vi "LDA_BSA_Comms_F60.vi"(2 "LDA Channels":T1[](array[typedef]) {"Sync Delay (s)" format="%.2g"; "Req Sampling Rate Hz" min=1.0; "Shifted mW" format="%.1g"; "Unshifted mW" format="%.1g"; "Centre Velocity (m/s)" format="%.2g"; "Velocity Range (m/s)" format="%.2g"; "Focal Length (mm)" format="%.1f"; "Beam Separation (mm)" format="%.1f"; "Optics Conversion Factor" format="%.3g"; "High voltage" min=0 max=2040 step=8; "Signal gain (dB)" min=0 max=30 step=1; "Min Velocity" format="%.2g"; "Max Velocity" format="%.2g"; "Wavelength (nm)" format="%.1f"}, 3 "BSA":refnum<k7>) -> (0 "error out":errorcluster, 1 "LDA Raw Data":cluster{dbl[][]}[](array[cluster]))   [LabVIEW 2021]
uses:
  LDA_Channel.ctl
  Globals/Meas_global.vi
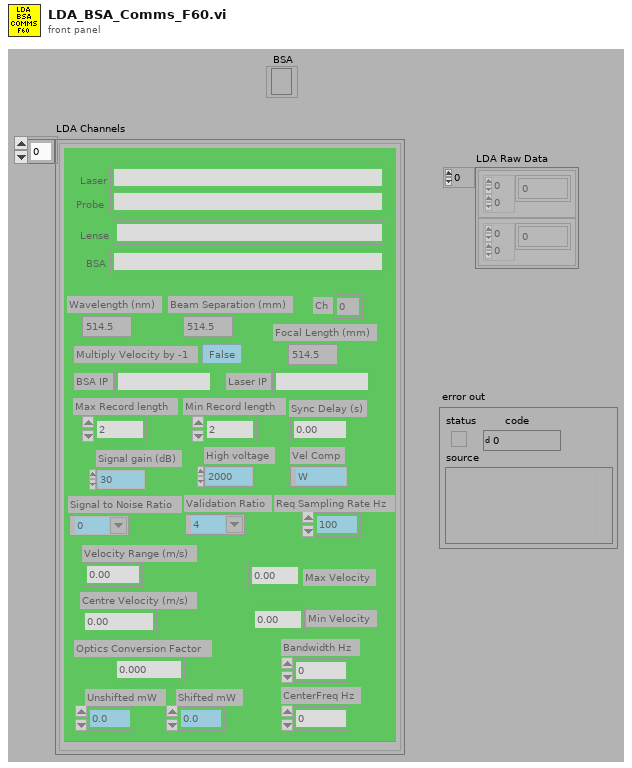
[diagram p1: front panel]
types:
  T1 = typedef "LDA_Channel.ctl" = cluster{"Wavelength (nm)":dbl, "Vel Comp":string, "Max Velocity":dbl, "Min Velocity":dbl, "Max Record length":u16, "Signal gain (dB)":i16, "High voltage":i16, "Optics Conversion Factor":dbl, "Min Record length":u16, "Multiply Velocity by -1":bool, "Signal to Noise Ratio":string, "Validation Ratio":string, "Probe":string, "Laser":string, "BSA":string, "Lense":string, "Beam Separation (mm)":dbl, "Focal Length (mm)":dbl, "COLOUR":u32, "BSA IP":string, "Velocity Range (m/s)":dbl, "Centre Velocity (m/s)":dbl, "Unshifted mW":dbl, "Shifted mW":dbl, "Bandwidth Hz":dbl, "Req Sampling Rate Hz":dbl, "Ch":i32, "CenterFreq Hz":dbl, "Laser IP":string, "Sync Delay (s)":dbl}
  T2 = typedef "Analysis_info_cluster.ctl" = cluster{"Colour":u32, "Inst type":T3, "Inst name":string, "Symbol":string, "Code name":string, "Extra Info":string, "Inst Array":T4, "Extra Titles":string[], "Extra Values":string[], "U":dbl, "u^2":dbl, "u^3":dbl, "u^4":dbl, "Skew_u":dbl, "Kurt_u":dbl, "Sd Error in Mean":dbl, "% u'/U":dbl, "X":dbl, "Y":dbl, "Z":dbl, "Timescale integral Estimate":dbl, "Sd Error in Variance":dbl, "Calib File":path, "Calib Constants":dbl[], "Output Position":bool, "Stats":enum16{"None", "Basic", "Full"}, "Av Sampling Rate":dbl, "Av No of Samples":dbl, "Total Meas Time (s)":dbl, "ADAM Ch Name":string, "Max value":dbl, "Min value":dbl, "Req Sample Rate Hz":dbl, "Sync Delay Time (s)":dbl, "Ch No":i16, "Device":string, "Use Latest Calib":bool, "Port":string, "Metadata Ch Names":string[], "Metadata Ch Values":string[], "Label":string}
  T3 = typedef "Inst_type.ctl" = enum16{"Raw voltage", "Raw with zero offsetting", "Propeller anemometer", "Pressure Transducer", "Pitot-static tube", "Hot wire", "Cross wire 1", "Cross wire 2", "Generic Linear", "Generic Polynomial", "Generic BackPoly", "Fast FID", "Thermocouple", "Cold wire", "Pulsed Wire", "LDA Vel", "LDA Tran time", "LDA Arr time", "Microphone"}
  T4 = typedef "Instrument_Array.ctl" = enum16{"PWA", "LDA", "Analogue"}
  T5 = typedef "Trigger_Mode.ctl" = enum16{"Free Running", "Start on Trigger", "Trigger Every Block", "Trigger Every Sample"}
  T6 = typedef "Rendezvous RefNum" = refnum<k1>
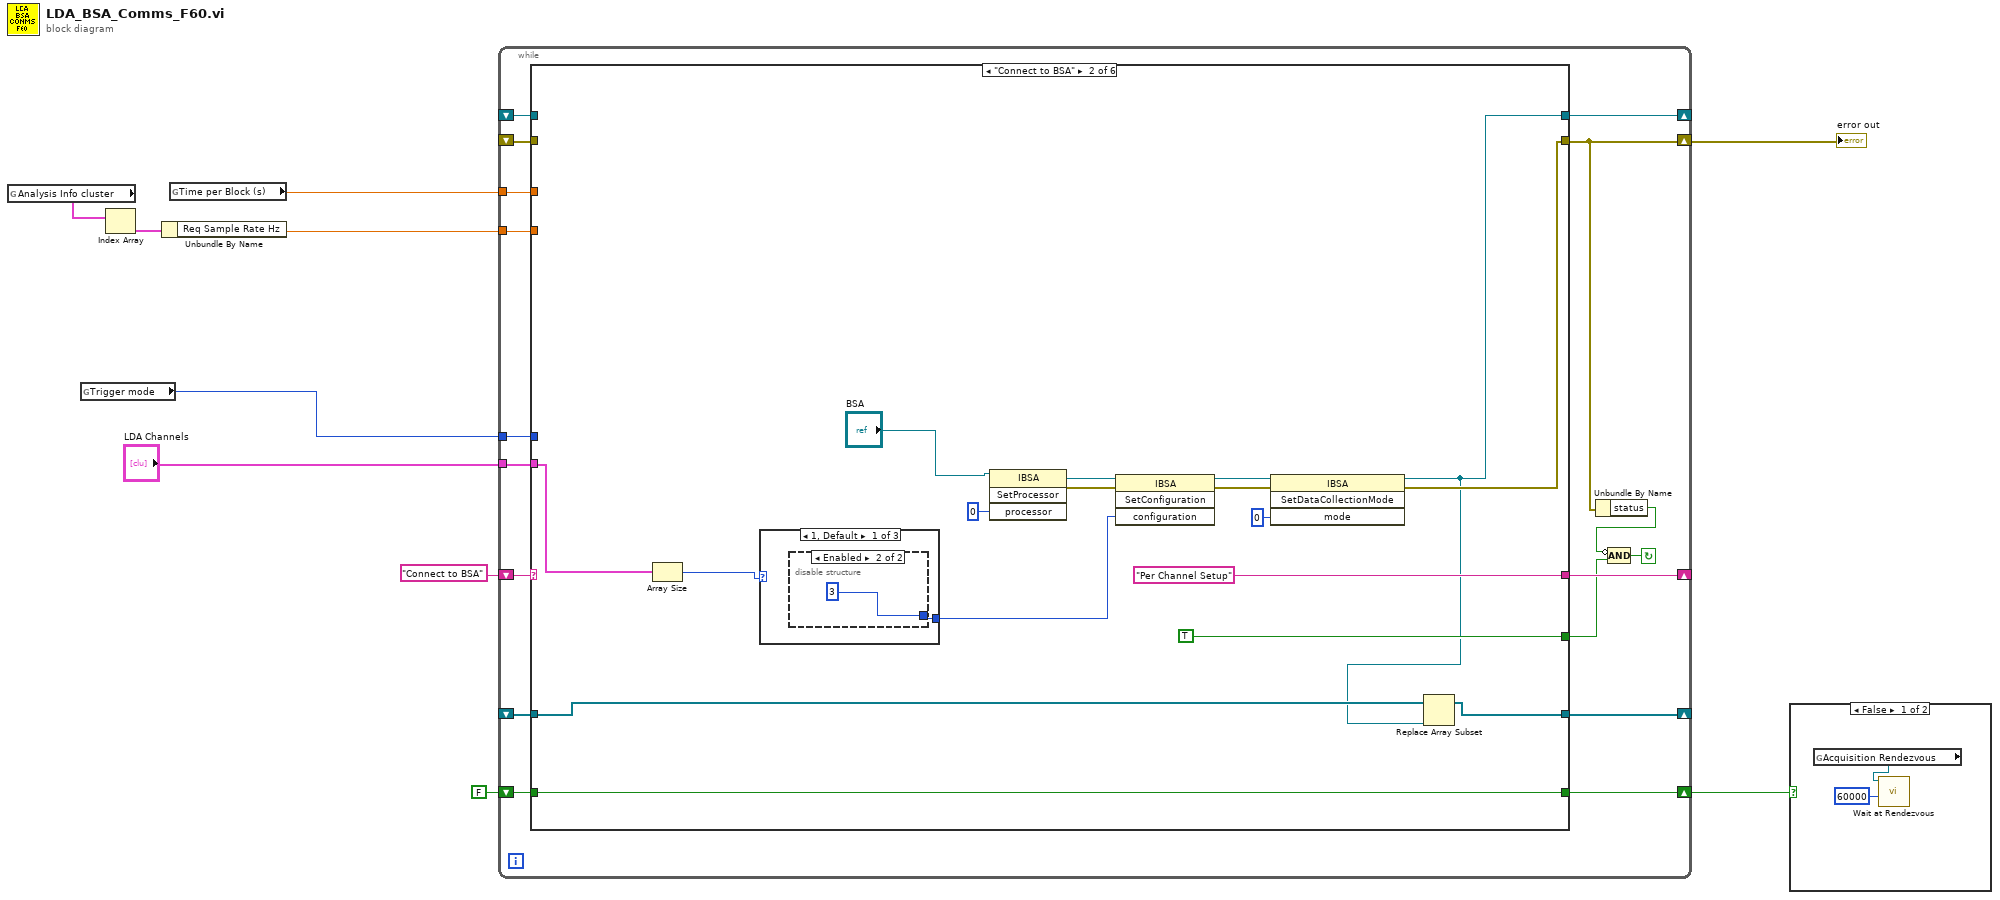
[diagram p0: block diagram]
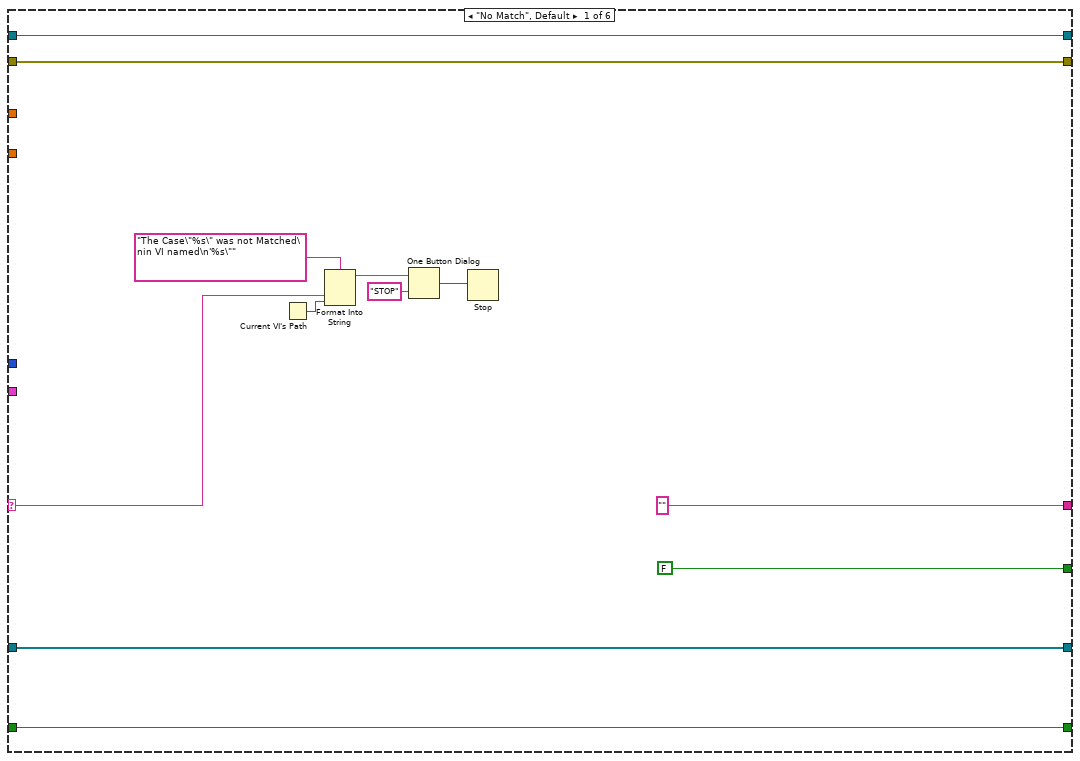
[diagram p2: hidden frame]
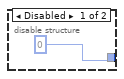
[diagram p3: hidden frame]
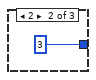
[diagram p4: hidden frame]
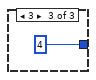
[diagram p5: hidden frame]
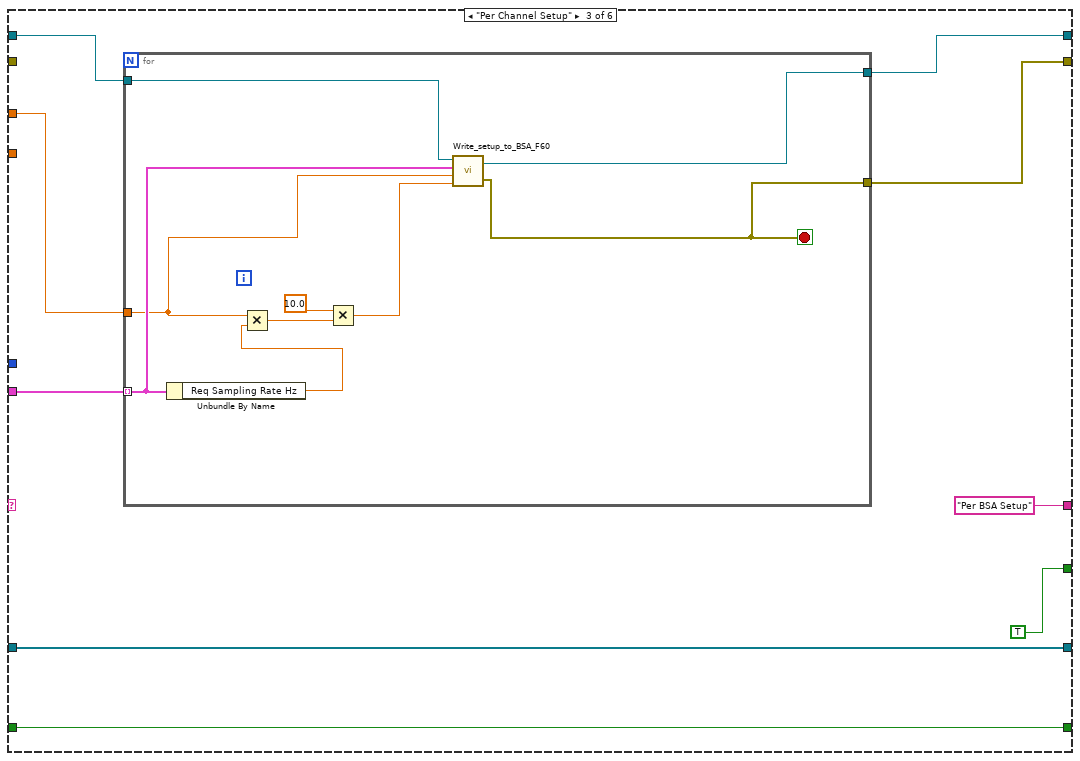
[diagram p6: hidden frame]
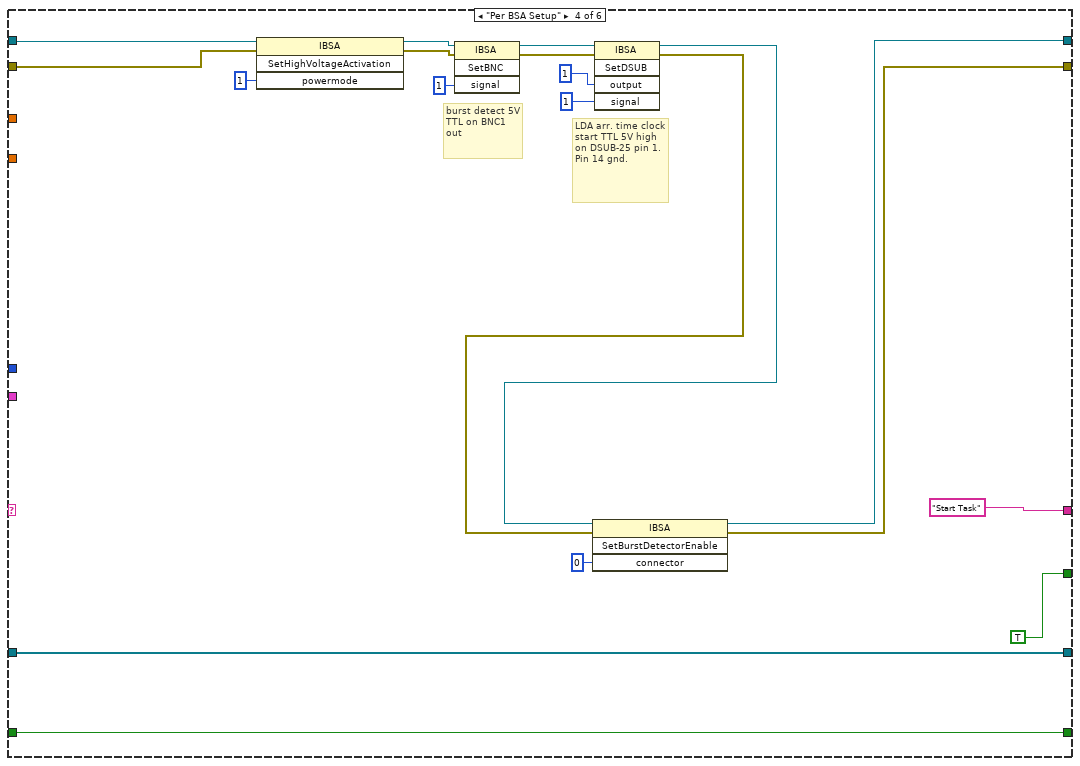
[diagram p7: hidden frame]
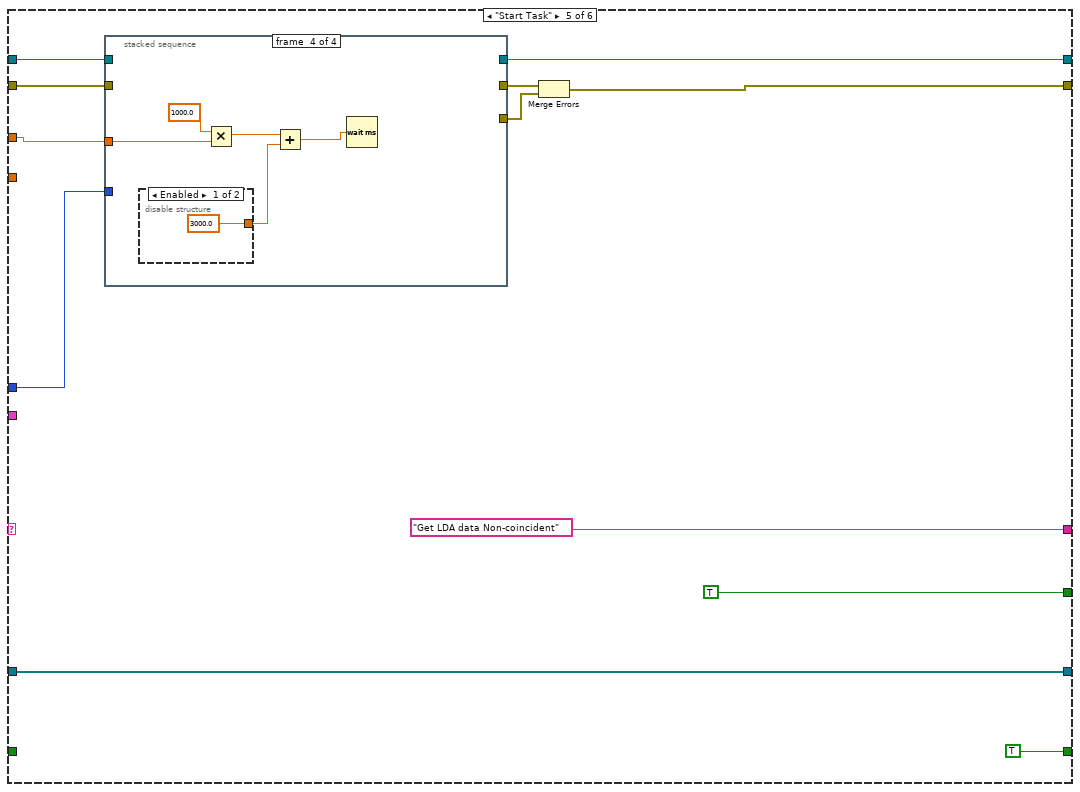
[diagram p8: hidden frame]
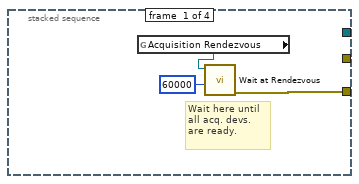
[diagram p9: hidden frame]
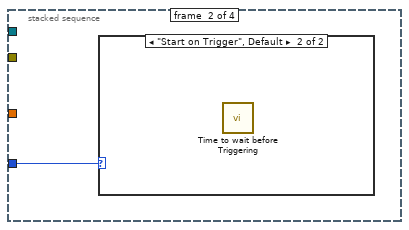
[diagram p10: hidden frame]
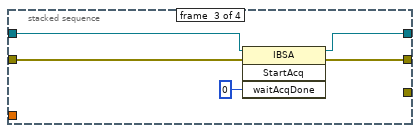
[diagram p12: hidden frame]
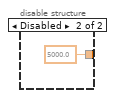
[diagram p13: hidden frame]
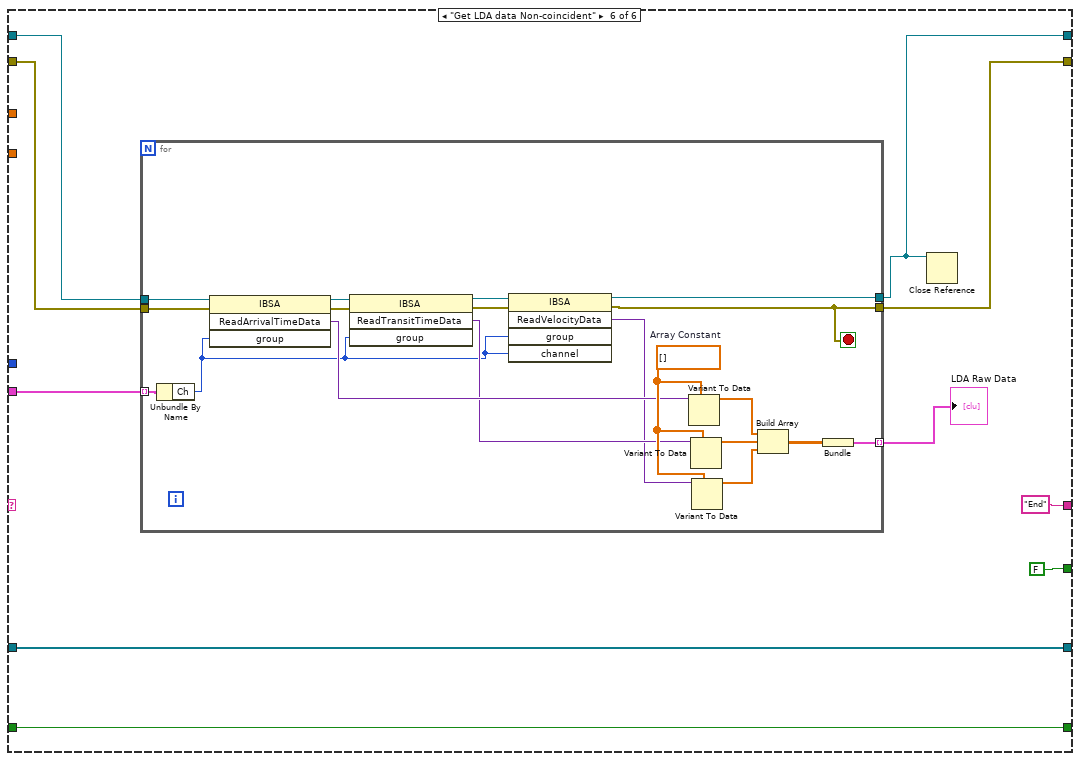
[diagram p14: hidden frame]
diagram:
  n1 = global read "Meas_global.vi" "Analysis Info cluster"() -> (w9:T2[])
  n2 = global read "Meas_global.vi" "Trigger mode"() -> (w5:T5)
  n3 = Index Array(array=w9) -> (element=w8:T2)  [unwired: 1 in]
  n4 = Unbundle By Name(w8) -> ("Req Sample Rate Hz"=w7:dbl)
  n5 = global read "Meas_global.vi" "Time per Block (s)"() -> (w6:dbl)
  n6 = while {
    shift-left: "Connect to BSA" -> [w26]
    shift-right: [w27] -> _
    shift-right: [w23] -> w10
    shift-left: _ -> [w16]
    tunnel: w7 -> [w25]
    shift-right: [w24] -> _
    shift-left: _ -> [w17]
    tunnel: w6 -> [w19]
    tunnel: w5 -> [w18]
    tunnel: "LDA Channels" -> [w15]
    shift-right: [w14] -> w4
    shift-left: FALSE -> [w13]
    shift-right: [w11] -> _
    shift-left: _ -> [w12]
    stop <- w21 continue-if-true
    n7 = case shown="\"Connect to BSA\"" w26 {
      selector: w26 -> [w30 _ _ _ _ _]
      tunnel: [FALSE TRUE TRUE TRUE TRUE FALSE] -> w20
      tunnel: ["" "Per Channel Setup" "Per BSA Setup" "Start Task" "Get LDA data Non-coincident" "End"] -> w27
      tunnel: [w32 w48 w64 w93 w105 w132] -> w23
      tunnel: w16 -> [w32 _ _ w96 w103 w135]
      tunnel: w25 -> [_ _ _ _ _ _]
      tunnel: w17 -> [w31 _ w66 w97 w104 w136]
      tunnel: [w31 w45 w65 w94 w109 w127] -> w24
      tunnel: w19 -> [_ _ w69 _ w99 _]
      tunnel: w18 -> [_ _ _ _ w102 _]
      tunnel: w15 -> [_ w42 w67 _ _ w131]
      tunnel: [w29 w47 w63 w81 TRUE w130] -> w14
      tunnel: w13 -> [w29 w47 w63 w81 _ w130]
      tunnel: w12 -> [w28 w46 w62 w80 w100 w129]
      tunnel: [w28 w44 w62 w80 w100 w129] -> w11
      frame "No Match", Default {
        n8 = Current VI's Path() -> (path=w34:path)
        n9 = Format Into String(format string="The Case\"%s\" was not Matched\nin VI named\n'%s\"" ("Format String"), w30, w34) -> (resulting string=w37:string)  [unwired: 2 in, 1 out]
        n10 = One Button Dialog(message=w37, button name ("OK")="STOP") -> (true=w35:bool)
        n11 = Stop(stop? (T)=w35) -> ()
      }
      frame "Connect to BSA" {
        n12 = Array Size(array=w42) -> (size(s)=w41:i32)
        n13 = case shown="1, Default" w41 {
          tunnel: [w57 3 ("configuration") 4 ("configuration")] -> w40
          frame 1, Default {
            n14 = disable-structure shown="Enabled" {
              disable-tunnel: [0 ("configuration") 3 ("configuration")] -> w57
              frame Disabled {
              }
              frame Enabled {
              }
            }
          }
          frame 2 {
          }
          frame 3 {
          }
        }
        n15 = invoke class="IBSA" method="SetProcessor"(reference="BSA", "processor"=0) -> (reference out=w53:refnum<k7>, error out=w52:errorcluster)  [unwired: 2 in, 2 out]
        n16 = invoke class="IBSA" method="SetConfiguration"(reference=w53, error in=w52, "configuration"=w40) -> (reference out=w51:refnum<k7>, error out=w50:errorcluster)  [unwired: 1 in, 2 out]
        n17 = invoke class="IBSA" method="SetDataCollectionMode"(reference=w51, error in=w50, "mode"=0) -> (reference out=w45:refnum<k7>, error out=w48:errorcluster)  [unwired: 1 in, 2 out]
        n18 = Replace Array Subset(array=w46, new element=w45) -> (w44:refnum<k7>[])  [unwired: 1 in]
      }
      frame "Per Channel Setup" {
        n19 = for {
          tunnel: w69 -> [w74]
          tunnel: w67 -> [w75] mode=indexing
          tunnel: w66 -> [w76]
          tunnel: [w72] -> w65
          tunnel: [w71] -> w64
          stop <- w71 stop-if-true
          n20 = Unbundle By Name(w75) -> ("Req Sampling Rate Hz"=w77:dbl)
          n21 = Multiply(x=w74, y=w77) -> (x*y=w78:dbl)
          n22 = Multiply(x=10.0 ("y"), y=w78) -> (x*y=w73:dbl)
          n23 = call "Write_setup_to_BSA_F60.vi"("No Of Samples"=w73, "Time (s)"=w74, "BSA Setup In"=w75, "BSA"=w76) -> ("error out"=w71:errorcluster, "reference out"=w72:refnum<k7>)
        }
      }
      frame "Per BSA Setup" {
        # "LDA arr. time clock start TTL 5V high on DSUB-25 pin 1. Pin 14 gnd."
        # "burst detect 5V TTL on BNC1 out"
        n24 = invoke class="IBSA" method="SetHighVoltageActivation"(reference=w97, error in=w96, "powermode"=1) -> (reference out=w85:refnum<k7>, error out=w84:errorcluster)  [unwired: 1 in, 2 out]
        n25 = invoke class="IBSA" method="SetBNC"(reference=w85, error in=w84, "signal"=1) -> (reference out=w92:refnum<k7>, error out=w91:errorcluster)  [unwired: 1 in, 2 out]
        n26 = invoke class="IBSA" method="SetDSUB"(reference=w92, error in=w91, "output"=1 ("signal"), "signal"=1) -> (reference out=w83:refnum<k7>, error out=w82:errorcluster)  [unwired: 1 in, 3 out]
        n27 = invoke class="IBSA" method="SetBurstDetectorEnable"(reference=w83, error in=w82, "connector"=0) -> (reference out=w94:refnum<k7>, error out=w93:errorcluster)  [unwired: 1 in, 2 out]
      }
      frame "Start Task" {
        n28 = stacked-sequence {
          tunnel: [_ _ w116 _] -> w107
          tunnel: w104 -> [_ _ w117 _]
          tunnel: [_ _ w115 _] -> w109
          tunnel: w103 -> [_ _ w118 _]
          tunnel: [w112 _ _ _] -> w106
          tunnel: w102 -> [_ w114 _ _]
          tunnel: w99 -> [_ _ _ w124]
          frame #0 {
            # "Wait here until all acq. devs. are ready."
            n29 = global read "Meas_global.vi" "Acquisition Rendezvous"() -> (w113:T6)
            n30 = call <vilib>:"Wait at Rendezvous.vi"("ms timeout (-1)"=60000, "rendezvous"=w113) -> ("error out"=w112:errorcluster)  [unwired: 3 in, 2 out]
          }
          frame #1 {
            n31 = case shown="\"Start on Trigger\", Default" w114 {
              frame "Free Running" {
              }
              frame "Start on Trigger", Default {
                n32 = call "Time to wait before Triggering.vi"() -> ()  [unwired: 12 in]
              }
            }
          }
          frame #2 {
            n33 = invoke class="IBSA" method="StartAcq"(reference=w117, error in=w118, "waitAcqDone"=0) -> (reference out=w115:refnum<k7>, error out=w116:errorcluster)  [unwired: 1 in, 2 out]
          }
          frame #3 {
            n34 = disable-structure shown="Enabled" {
              disable-tunnel: [3000.0 ("y") 5000.0 ("y")] -> w121
              frame Enabled {
              }
              frame Disabled {
              }
            }
            n35 = Multiply(x=1000.0, y=w124) -> (x*y=w122:dbl)
            n36 = Add(x=w122, y=w121) -> (x+y=w120:dbl)
            n37 = Wait (ms)(milliseconds to wait=w120) -> ()  [unwired: 1 out]
          }
        }
        n38 = Merge Errors(w107, w106) -> (w105:errorcluster)
      }
      frame "Get LDA data Non-coincident" {
        n39 = for {
          tunnel: w136 -> [w147]
          tunnel: w135 -> [w146]
          tunnel: [w141] -> w128 mode=indexing
          tunnel: [w140] -> w127
          tunnel: [w139] -> w132
          tunnel: w131 -> [w138] mode=indexing
          stop <- w139 stop-if-true
          w151 = dbl[] []  # Array Constant
          n40 = Unbundle By Name(w138) -> ("Ch"=w137:i32)
          n41 = invoke class="IBSA" method="ReadArrivalTimeData"(reference=w147, error in=w146, "group"=w137) -> (reference out=w155:refnum<k7>, error out=w154:errorcluster, "ReadArrivalTimeData"=w150:variant)  [unwired: 1 in, 1 out]
          n42 = invoke class="IBSA" method="ReadTransitTimeData"(reference=w155, error in=w154, "group"=w137) -> (reference out=w153:refnum<k7>, error out=w152:errorcluster, "ReadTransitTimeData"=w149:variant)  [unwired: 1 in, 1 out]
          n43 = invoke class="IBSA" method="ReadVelocityData"(reference=w153, error in=w152, "group"=w137, "channel"=w137) -> (reference out=w140:refnum<k7>, error out=w139:errorcluster, "ReadVelocityData"=w148:variant)  [unwired: 1 in, 2 out]
          n44 = Variant To Data(type=w151, Variant=w150) -> (data=w145:dbl[])  [unwired: 1 in, 1 out]
          n45 = Variant To Data(type=w151, Variant=w149) -> (data=w144:dbl[])  [unwired: 1 in, 1 out]
          n46 = Variant To Data(type=w151, Variant=w148) -> (data=w143:dbl[])  [unwired: 1 in, 1 out]
          n47 = Build Array(w145, w144, w143) -> (w142:dbl[][])
          n48 = Bundle(w142) -> (w141:cluster{dbl[][]})  [unwired: 1 in]
        }
        "LDA Raw Data" <- w128
        n49 = Close Reference(reference=w127) -> ()  [unwired: 1 in, 1 out]
      }
    }
    n50 = Unbundle By Name(w23) -> ("status"=w22:bool)
    n51 = Compound Arithmetic op=AND(invert w22, w20) -> (w21:bool)
  }
  "error out" <- w10
  n52 = case shown="False" w4 {
    frame False {
      n53 = global read "Meas_global.vi" "Acquisition Rendezvous"() -> (w156:T6)
      n54 = call <vilib>:"Wait at Rendezvous.vi"("ms timeout (-1)"=60000, "rendezvous"=w156) -> ()  [unwired: 3 in, 3 out]
    }
    frame True {
    }
  }
